vi "Invoke Measure Logic.vi"(8 "error in":errorcluster, 10 "gRPCid in":T1, 11 "gRPC Server in":refnum<class "MeasurementPluginService.lvclass">) -> (0 "error out":errorcluster)   [LabVIEW 2020, in "MeasurementLink Measurement Server.lvlib" / "MeasurementPluginService.lvclass"]
uses:
  MeasurementPluginService.lvclass
  <vilib>/gRPC/LabVIEW gRPC Library/Shared/grpcId.ctl
  MeasurementContext/MeasurementContext.lvclass
  MeasurementLink Measurement Server Internal/RPC Service/MeasurementService/MeasurementService.lvclass
  <vilib>/gRPC/LabVIEW gRPC Library/grpc-lvsupport-release.lvlib
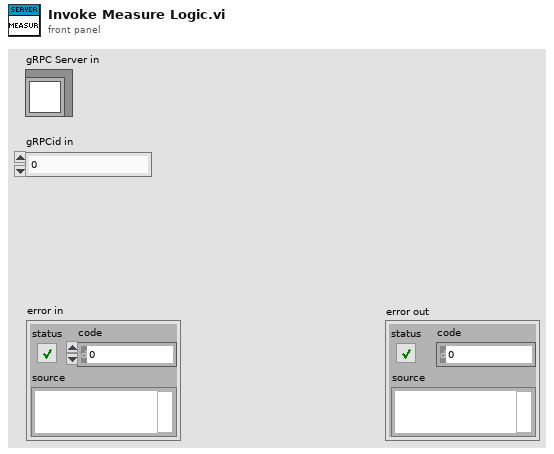
[diagram p1: front panel]
types:
  T1 = typedef "grpc-lvsupport-release.lvlib/grpcId.ctl" = u64
  T2 = typedef "MeasurementLink Measurement Server Internal.lvlib/ni_measurementlink_measurement_v1_MeasureRequest.ctl" = cluster{"configuration_parameters":T3, "pin_map_context":T4}
  T3 = typedef "MeasurementLink Measurement Server Internal.lvlib/google_protobuf_Any.ctl" = cluster{"type_url":string, "value":u8[]}
  T4 = typedef "MeasurementLink Measurement Server Internal.lvlib/ni_measurementlink_PinMapContext.ctl" = cluster{"pin_map_id":string, "sites":i32[]}
  T5 = typedef "grpc-lvsupport-release.lvlib/Any.ctl" = cluster{"Type Url":string, "Bytes":u8[]}
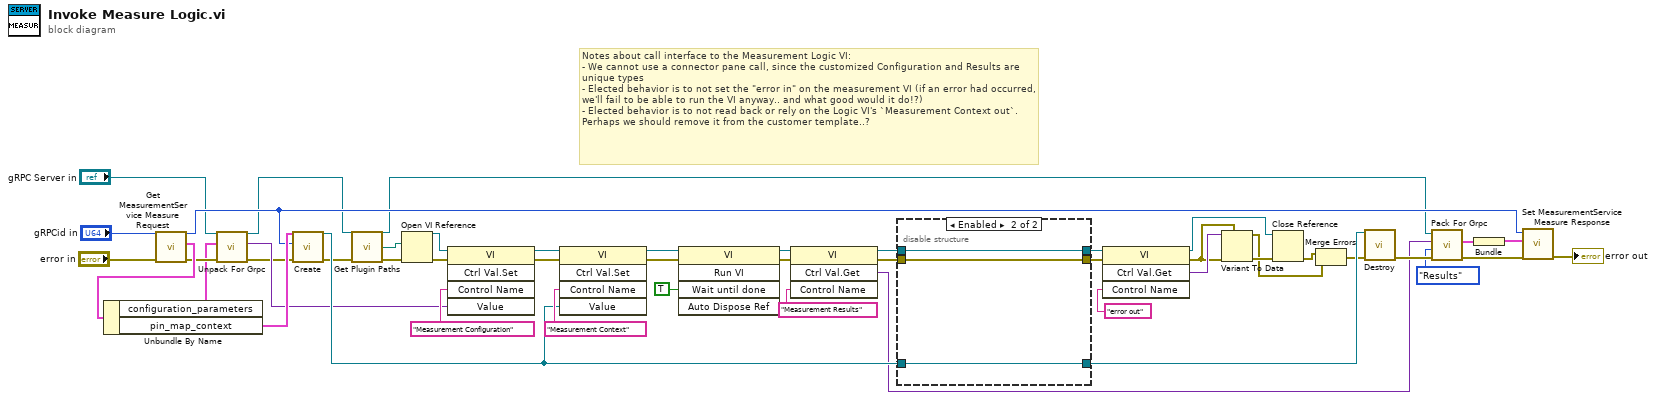
[diagram p0: block diagram]
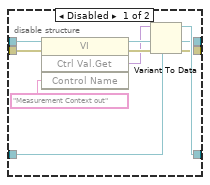
[diagram p2: hidden frame]
diagram:
  # "Notes about call interface to the Measurement Logic VI:\n- We cannot use a connector pane call, since the customized Configuration and Results are unique types\n- Elected behavior is to not set the \"error in\" on the measurement VI (if an error had occurred, we'll fail to be able to run the VI anyway.. and what good would it do!?)\n- Elected behavior is to not read back or rely on the Logic VI's `Measurement Context out`.  Perhaps we should remove it from the customer template..?"
  n1 = call "Get MeasurementService Measure Request.vi"("error in (no error)"="error in", "gRPCid in"="gRPCid in") -> ("error out"=w20:errorcluster, "Message Data"=w48:T2, "gRPCid out"=w21:T1)  [unwired: 7 in]
  n2 = Unbundle By Name(w48) -> ("configuration_parameters"=w11:T3, "pin_map_context"=w47:T4)
  n3 = call-dynamic "Unpack For Grpc.vi"("error in (no error)"=w20, "Any"=w11, "gRPC Server in"="gRPC Server in") -> ("error out"=w18:errorcluster, "Data Value"=w19:variant, "gRPC Server out"=w10:refnum<class "MeasurementPluginService.lvclass">)  [unwired: 6 in]
  n4 = call "Create.vi"("error in (no error)"=w18, "gRPC server call"=w21, "pin map context"=w47) -> ("error out"=w14:errorcluster, "MeasurementContext out"=w33:refnum<class "MeasurementContext.lvclass">)  [unwired: 7 in]
  n5 = call-dynamic "Get Plugin Paths.vi"("MeasurementService in"=w10, "error in (no error)"=w14) -> ("MeasurementService out"=w6:refnum<class "MeasurementPluginService.lvclass">, "Measurement Logic VI Path"=w13:path, "error out"=w15:errorcluster)  [unwired: 7 in, 4 out]
  n6 = Open VI Reference(vi path=w13, error in (no error)=w15) -> (vi reference=w45:refnum<vi>, error out=w44:errorcluster)  [unwired: 4 in]
  n7 = invoke class="VI" method="Ctrl Val.Set"(reference=w45, error in=w44, "Control Name"="Measurement Configuration", "Value"=w19) -> (reference out=w42:refnum<vi>, error out=w41:errorcluster)  [unwired: 1 in, 3 out]
  n8 = invoke class="VI" method="Ctrl Val.Set"(reference=w42, error in=w41, "Control Name"="Measurement Context", "Value"=w33) -> (reference out=w38:refnum<vi>, error out=w39:errorcluster)  [unwired: 1 in, 3 out]
  n9 = invoke class="VI" method="Run VI"(reference=w38, error in=w39, "Wait until done"=TRUE ("Wait Until Done")) -> (reference out=w36:refnum<vi>, error out=w35:errorcluster)  [unwired: 2 in, 3 out]
  n10 = invoke class="VI" method="Ctrl Val.Get"(reference=w36, error in=w35, "Control Name"="Measurement Results") -> (reference out=w31:refnum<vi>, error out=w22:errorcluster, "Get Control Value Variant"=w7:variant)  [unwired: 1 in, 1 out]
  n11 = disable-structure shown="Enabled" {
    disable-tunnel: w33 -> [w57 w60]
    disable-tunnel: [w56 w60] -> w32
    disable-tunnel: w31 -> [w55 w58]
    disable-tunnel: [w54 w58] -> w30
    disable-tunnel: [w53 w59] -> w29
    disable-tunnel: w22 -> [w52 w59]
    frame Disabled {
      n12 = invoke class="VI" method="Ctrl Val.Get"(reference=w55, error in=w52, "Control Name"="Measurement Context out") -> (reference out=w54:refnum<vi>, error out=w50:errorcluster, "Get Control Value Variant"=w49:variant)  [unwired: 1 in, 1 out]
      n13 = Variant To Data(error in=w50, type=w57, Variant=w49) -> (data=w56:refnum<class "MeasurementContext.lvclass">, error out=w53:errorcluster)
    }
    frame Enabled {
    }
  }
  n14 = invoke class="VI" method="Ctrl Val.Get"(reference=w30, error in=w29, "Control Name"="error out") -> (reference out=w26:refnum<vi>, error out=w25:errorcluster, "Get Control Value Variant"=w27:variant)  [unwired: 1 in, 1 out]
  n15 = Variant To Data(error in=w25, type=w25, Variant=w27) -> (data=w23:errorcluster, error out=w24:errorcluster)
  n16 = Close Reference(reference=w26, error in (no error)=w24) -> (error out=w46:errorcluster)
  n17 = Merge Errors(w46, w23) -> (w9:errorcluster)
  n18 = call-dynamic "Destroy.vi"("error in (no error)"=w9, "MeasurementContext in"=w32) -> ("error out"=w8:errorcluster)  [unwired: 9 in]
  n19 = call-dynamic "Pack For Grpc.vi"("error in (no error)"=w8, "Configuration / Resuls (Config)"=enum16{"Configuration", "Results"}."Results", "Data Value"=w7, "gRPC Server in"=w6) -> ("error out"=w4:errorcluster, "Any"=w3:T5)  [unwired: 5 in, 1 out]
  n20 = Bundle("Any"=w3) -> (w2:cluster{"Any":T5})  [unwired: 1 in]
  n21 = call "Set MeasurementService Measure Response.vi"("error in (no error)"=w4, "Message Data"=w2, "gRPCid in"=w21) -> ("error out"=→"error out":errorcluster)  [unwired: 8 in]
